vi "Ejercicio 1 3.vi"() -> ()   [LabVIEW 2021]
panel:
  out "Código":string
  in  "stop":bool
  out "Señal":i32(graph)
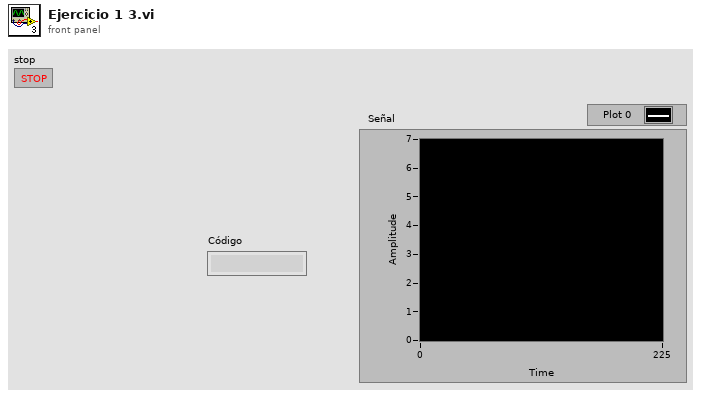
[diagram p1: front panel]
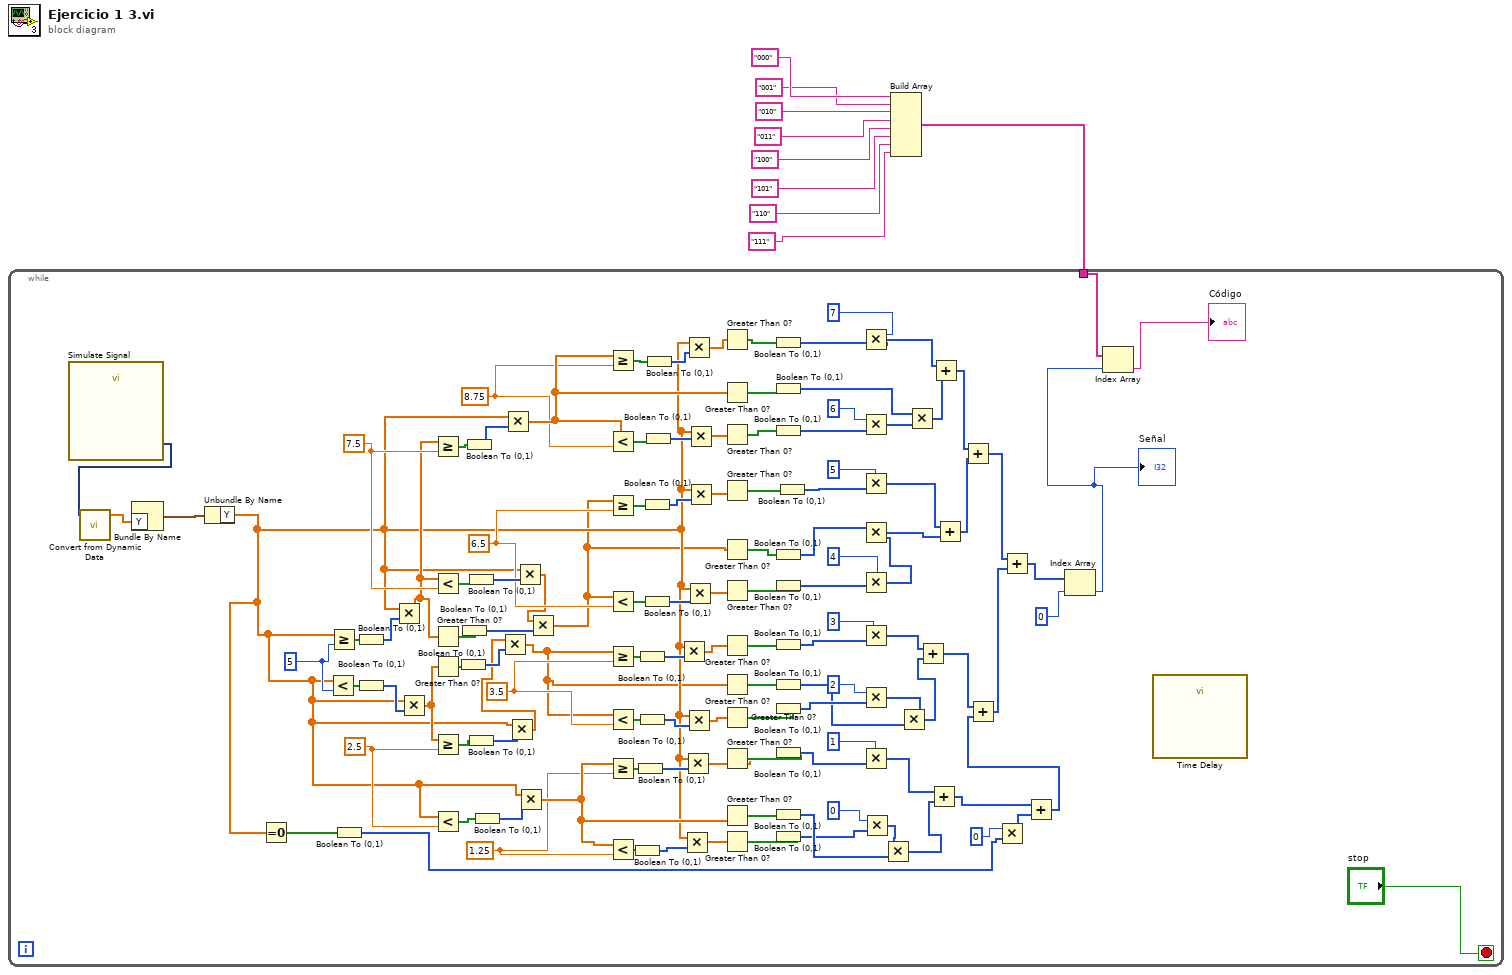
[diagram p0: block diagram]
diagram:
  n1 = Build Array("000", "001", "010", "011", "100", "101", "110", "111") -> (w9:string[])
  n2 = while {
    tunnel: w9 -> [w33]
    stop <- "stop" stop-if-true
    w38 = 3.5
    w39 = 1.25
    w40 = 2.5
    w36 = 6.5
    w37 = 8.75
    w35 = 7.5
    w34 = 5
    n3 = call "Simulate Signal"() -> ("Sine"=w129:dynamicdata)  [unwired: 14 in, 1 out]
    n4 = call "Convert from Dynamic Data"("Dynamic Data Type"=w129) -> ("Array"=w127:dbl[])  [unwired: 3 in]
    n5 = Bundle By Name("Y"=w127) -> (w128:waveform(dbl))  [unwired: 1 in]
    n6 = Unbundle By Name(w128) -> ("Y"=w20:dbl[])
    n7 = Equal To 0?(x=w20) -> (x = 0?=w109:bool[])
    n8 = Less?(x=w20, y=w34) -> (x < y?=w53:bool[])
    n9 = Greater Or Equal?(x=w20, y=w34) -> (x >= y?=w49:bool[])
    n10 = Boolean To (0,1)(Boolean=w109) -> (0, 1=w110:i16[])
    n11 = Boolean To (0,1)(Boolean=w49) -> (0, 1=w50:i16[])
    n12 = Boolean To (0,1)(Boolean=w53) -> (0, 1=w64:i16[])
    n13 = Multiply(x=w20, y=w50) -> (x*y=w29:dbl[])
    n14 = Multiply(x=w20, y=w64) -> (x*y=w28:dbl[])
    n15 = Greater Or Equal?(x=w29, y=w35) -> (x >= y?=w51:bool[])
    n16 = Less?(x=w29, y=w35) -> (x < y?=w54:bool[])
    n17 = Greater Than 0?(x=w29) -> (x > 0?=w27:bool[])
    n18 = Greater Than 0?(x=w28) -> (x > 0?=w26:bool[])
    n19 = Greater Or Equal?(x=w28, y=w40) -> (x >= y?=w76:bool[])
    n20 = Less?(x=w20, y=w40) -> (x < y?=w75:bool[])
    n21 = Boolean To (0,1)(Boolean=w26) -> (0, 1=w23:i16[])
    n22 = Boolean To (0,1)(Boolean=w27) -> (0, 1=w25:i16[])
    n23 = Boolean To (0,1)(Boolean=w51) -> (0, 1=w52:i16[])
    n24 = Boolean To (0,1)(Boolean=w54) -> (0, 1=w55:i16[])
    n25 = Boolean To (0,1)(Boolean=w76) -> (0, 1=w73:i16[])
    n26 = Boolean To (0,1)(Boolean=w75) -> (0, 1=w74:i16[])
    n27 = Multiply(x=w20, y=w52) -> (x*y=w119:dbl[])
    n28 = Multiply(x=w20, y=w73) -> (x*y=w22:dbl[])
    n29 = Multiply(x=w22, y=w23) -> (x*y=w15:dbl[])
    n30 = Multiply(x=w20, y=w55) -> (x*y=w24:dbl[])
    n31 = Multiply(x=w20, y=w74) -> (x*y=w104:dbl[])
    n32 = Multiply(x=w24, y=w25) -> (x*y=w13:dbl[])
    n33 = Greater Or Equal?(x=w119, y=w37) -> (x >= y?=w56:bool[])
    n34 = Less?(x=w119, y=w37) -> (x < y?=w58:bool[])
    n35 = Greater Or Equal?(x=w13, y=w36) -> (x >= y?=w60:bool[])
    n36 = Less?(x=w13, y=w36) -> (x < y?=w61:bool[])
    n37 = Greater Or Equal?(x=w15, y=w38) -> (x >= y?=w72:bool[])
    n38 = Less?(x=w15, y=w38) -> (x < y?=w70:bool[])
    n39 = Greater Or Equal?(x=w104, y=w39) -> (x >= y?=w67:bool[])
    n40 = Less?(x=w104, y=w39) -> (x < y?=w65:bool[])
    n41 = Boolean To (0,1)(Boolean=w65) -> (0, 1=w66:i16[])
    n42 = Boolean To (0,1)(Boolean=w67) -> (0, 1=w68:i16[])
    n43 = Boolean To (0,1)(Boolean=w72) -> (0, 1=w71:i16[])
    n44 = Boolean To (0,1)(Boolean=w70) -> (0, 1=w69:i16[])
    n45 = Boolean To (0,1)(Boolean=w60) -> (0, 1=w62:i16[])
    n46 = Boolean To (0,1)(Boolean=w61) -> (0, 1=w63:i16[])
    n47 = Boolean To (0,1)(Boolean=w58) -> (0, 1=w59:i16[])
    n48 = Boolean To (0,1)(Boolean=w56) -> (0, 1=w57:i16[])
    n49 = Multiply(x=w20, y=w71) -> (x*y=w16:dbl[])
    n50 = Multiply(x=w20, y=w66) -> (x*y=w83:dbl[])
    n51 = Multiply(x=w20, y=w68) -> (x*y=w82:dbl[])
    n52 = Multiply(x=w20, y=w57) -> (x*y=w77:dbl[])
    n53 = Multiply(x=w20, y=w69) -> (x*y=w81:dbl[])
    n54 = Multiply(x=w20, y=w63) -> (x*y=w80:dbl[])
    n55 = Multiply(x=w20, y=w59) -> (x*y=w78:dbl[])
    n56 = Multiply(x=w20, y=w62) -> (x*y=w79:dbl[])
    n57 = Greater Than 0?(x=w77) -> (x > 0?=w84:bool[])
    n58 = Greater Than 0?(x=w119) -> (x > 0?=w120:bool[])
    n59 = Greater Than 0?(x=w78) -> (x > 0?=w17:bool[])
    n60 = Greater Than 0?(x=w79) -> (x > 0?=w90:bool[])
    n61 = Greater Than 0?(x=w13) -> (x > 0?=w121:bool[])
    n62 = Greater Than 0?(x=w80) -> (x > 0?=w89:bool[])
    n63 = Greater Than 0?(x=w16) -> (x > 0?=w88:bool[])
    n64 = Greater Than 0?(x=w15) -> (x > 0?=w114:bool[])
    n65 = Greater Than 0?(x=w81) -> (x > 0?=w87:bool[])
    n66 = Greater Than 0?(x=w82) -> (x > 0?=w86:bool[])
    n67 = Greater Than 0?(x=w104) -> (x > 0?=w105:bool[])
    n68 = Greater Than 0?(x=w83) -> (x > 0?=w85:bool[])
    n69 = Boolean To (0,1)(Boolean=w84) -> (0, 1=w91:i16[])
    n70 = Boolean To (0,1)(Boolean=w120) -> (0, 1=w14:i16[])
    n71 = Boolean To (0,1)(Boolean=w17) -> (0, 1=w97:i16[])
    n72 = Boolean To (0,1)(Boolean=w121) -> (0, 1=w124:i16[])
    n73 = Boolean To (0,1)(Boolean=w89) -> (0, 1=w95:i16[])
    n74 = Boolean To (0,1)(Boolean=w88) -> (0, 1=w94:i16[])
    n75 = Boolean To (0,1)(Boolean=w114) -> (0, 1=w116:i16[])
    n76 = Boolean To (0,1)(Boolean=w87) -> (0, 1=w117:i16[])
    n77 = Boolean To (0,1)(Boolean=w86) -> (0, 1=w93:i16[])
    n78 = Boolean To (0,1)(Boolean=w105) -> (0, 1=w106:i16[])
    n79 = Boolean To (0,1)(Boolean=w85) -> (0, 1=w92:i16[])
    n80 = Boolean To (0,1)(Boolean=w90) -> (0, 1=w96:i16[])
    n81 = Multiply(x=7, y=w91) -> (x*y=w98:i32[])
    n82 = Multiply(x=6, y=w97) -> (x*y=w122:i32[])
    n83 = Multiply(x=5, y=w96) -> (x*y=w99:i32[])
    n84 = Multiply(x=4, y=w95) -> (x*y=w125:i32[])
    n85 = Multiply(x=w124, y=w125) -> (x*y=w126:i32[])
    n86 = Multiply(x=3, y=w94) -> (x*y=w100:i32[])
    n87 = Multiply(x=2, y=w117) -> (x*y=w115:i32[])
    n88 = Multiply(x=1, y=w93) -> (x*y=w101:i32[])
    n89 = Multiply(x=0, y=w92) -> (x*y=w107:i32[])
    n90 = Multiply(x=w107, y=w106) -> (x*y=w108:i32[])
    n91 = Multiply(x=w115, y=w116) -> (x*y=w118:i32[])
    n92 = Multiply(x=w14, y=w122) -> (x*y=w123:i32[])
    n93 = Add(x=w100, y=w118) -> (x+y=w103:i32[])
    n94 = Add(x=w101, y=w108) -> (x+y=w112:i32[])
    n95 = Add(x=w98, y=w123) -> (x+y=w30:i32[])
    n96 = Add(x=w99, y=w126) -> (x+y=w102:i32[])
    n97 = Add(x=w30, y=w102) -> (x+y=w21:i32[])
    n98 = Multiply(x=0, y=w110) -> (x*y=w111:i32[])
    n99 = Add(x=w112, y=w111) -> (x+y=w113:i32[])
    n100 = Add(x=w103, y=w113) -> (x+y=w31:i32[])
    n101 = Add(x=w21, y=w31) -> (x+y=w19:i32[])
    n102 = Index Array(array=w19, index=0) -> (element=w12:i32)
    "Señal" <- w12
    n103 = Index Array(array=w33, index=w12) -> (element=→"Código":string)
    n104 = call "Time Delay"() -> ()  [unwired: 11 in, 1 out]
  }
